vi "SUB_SW_Version.vi"() -> (1 "Current Software Version":string)   [LabVIEW 2011]
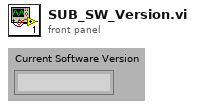
[diagram p1: front panel]
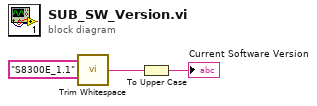
[diagram p0: block diagram]
diagram:
  n1 = call <vilib>:"Trim Whitespace.vi"("string"="S8300E_1.1") -> ("trimmed string"=w2:string)  [unwired: 1 in]
  n2 = To Upper Case(1:w2) -> (0:→"Current Software Version":string)
